vi "doma.vi"() -> ()   [LabVIEW 2017]
uses:
  <vilib>/userdefined/High Color/IMAQdx.ctl
  <vilib>/myRIO/Instrument Drivers/Onboard IO/DIO/typedefs/DIO Reference.ctl
  <vilib>/myRIO/Common/Instrument Driver Framework/Utilities/typedefs/myRIO Generic Hardware Reference.ctl
  <vilib>/myRIO/Common/Instrument Driver Framework/Utilities/typedefs/Hardware Version Enum.ctl
  <vilib>/myRIO/Common/Instrument Driver Framework/Utilities/typedefs/myRIO v1.0 Reference.ctl
  <vilib>/myRIO/Common/Instrument Driver Framework/Utilities/typedefs/Generic FPGA Reference.ctl
  <vilib>/myRIO/Common/Instrument Driver Framework/myRIO v1.0/DIO/typedefs/DIO Channels List.ctl
  <vilib>/myRIO/Common/Instrument Driver Framework/myRIO v1.0/DIO/typedefs/DIO Channels Enum.ctl
  <vilib>/userdefined/High Color/nirio_resource_hc.ctl
  <vilib>/myRIO/Common/Instrument Driver Framework/Utilities/vis/Is FPGA Ref Available.vi
  <vilib>/myRIO/Common/Instrument Driver Framework/myRIO v1.0/DIO/vis/myRIO v1.1 Open DIO.vi
  <vilib>/myRIO/Instrument Drivers/Onboard IO/DIO/vis/Write.vi
  <vilib>/myRIO/Common/Instrument Driver Framework/Utilities/vis/Validate Channels.vi
  <vilib>/myRIO/Common/Instrument Driver Framework/myRIO v1.0/DIO/vis/myRIO v1.0 Reserve DIO.vi
  <vilib>/myRIO/Common/Instrument Driver Framework/myRIO v1.0/Resource Manager/vis/myRIO v1.0 Reserve Channel List.vi
  <vilib>/myRIO/Common/Instrument Driver Framework/myRIO v1.0/DIO/vis/myRIO v1.0 Build MUX Configuration DIO.vi
  <vilib>/myRIO/Common/Instrument Driver Framework/myRIO v1.0/Resource Manager/vis/myRIO v1.0 Reserve Channel.vi
  <vilib>/myRIO/Common/Instrument Driver Framework/myRIO v1.0/Resource Manager/vis/myRIO v1.0 Unreserve Channel.vi
  <vilib>/myRIO/Common/Instrument Driver Framework/myRIO v1.0/Resource Manager/vis/myRIO v1.0 Create Configuration List.vi
  <vilib>/myRIO/Common/Instrument Driver Framework/myRIO v1.0/Resource Manager/vis/myRIO v1.0 Build Mutex Name.vi
  addres.vi
  <vilib>/Utility/VariantDataType/GetNumericInfo.vi
  <vilib>/Utility/error.llb/Error Cluster From Error Code.vi
  <vilib>/myRIO/Common/Instrument Driver Framework/myRIO v1.0/myRIO v1.1 Open.vi
  <vilib>/myRIO/Common/Instrument Driver Framework/Utilities/vis/IO Manager.vi
  <vilib>/myRIO/Common/Instrument Driver Framework/Utilities/vis/Configuration Manager.vi
  <vilib>/myRIO/Common/Instrument Driver Framework/myRIO v1.0/Resource Manager/vis/myRIO v1.0 Configure IO.vi
  <vilib>/myRIO/Common/Instrument Driver Framework/myRIO v1.0/myRIO v1.0 Close.vi
  <vilib>/myRIO/Common/Instrument Driver Framework/myRIO v1.0/DIO/vis/myRIO v1.0 Write DIO.vi
  <vilib>/myRIO/Express VI/Onboard Devices/LED/LED Express VI.xnode
  <vilib>/myRIO/Instrument Drivers/Onboard IO/DIO/vis/myRIO DIO Open.xnode
  <vilib>/vision/driver/NI_Vision_Acquisition_Software.lvlib
  <vilib>/myRIO/Instrument Drivers/Onboard IO/DIO/DIO.lvlib
panel:
  out "number":string
  out "color":string
  out "error out":errorcluster
  in  "error in":errorcluster
  out "Image":T1(plugin-control)
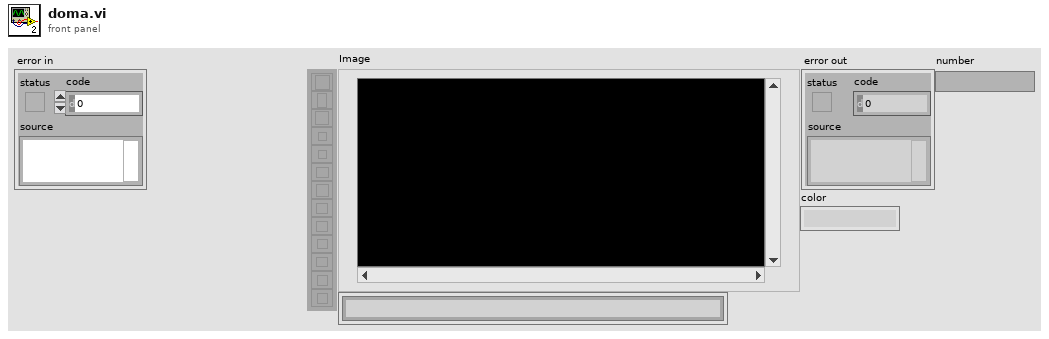
[diagram p1: front panel]
types:
  T1 = typedef "IMAQ Image.ctl" = refnum<image>
  T2 = typedef "IMAQdx.ctl" = refnum<k21>
  T3 = typedef "DIO.lvlib/DIO Reference.ctl" = cluster{"myRIO Reference":T4, "DIO Channels List":T8}
  T4 = typedef "myRIO Generic Hardware Reference.ctl" = cluster{"myRIO Model":T5, "myRIO Hardware Reference":T6}
  T5 = typedef "Hardware Version Enum.ctl" = enum16{"Unknown", "myRIO-1900", "myRIO-1950", "roboRIO", "NI ELVIS RIO CM"}
  T6 = typedef "myRIO v1.0 Reference.ctl" = cluster{"Generic FPGA Reference":T7, "Allow multiple opens":bool}
  T7 = typedef "Generic FPGA Reference.ctl" = refnum<k20>
  T8 = typedef "DIO Channels List.ctl" = T9[]
  T9 = typedef "DIO Channels Enum.ctl" = enum16{"Not Connected", "C/DIO0", "C/DIO1", "C/DIO2", "C/DIO3", "C/DIO4", "C/DIO5", "C/DIO6", "C/DIO7", "A/DIO0", "A/DIO1", "A/DIO2", "A/DIO3", "A/DIO4", "A/DIO5", "A/DIO6", "A/DIO7", "A/DIO8", "A/DIO9", "A/DIO10", "A/DIO11", "A/DIO12", "A/DIO13", "A/DIO14", "A/DIO15", "B/DIO0", "B/DIO1", "B/DIO2", "B/DIO3", "B/DIO4", "B/DIO5", "B/DIO6", "B/DIO7", "B/DIO8", "B/DIO9", "B/DIO10", "B/DIO11", "B/DIO12", "B/DIO13", "B/DIO14", "B/DIO15", "LED0", "LED1", "LED2", "LED3", "Button0", "DIO/DIO0", "DIO/DIO1", "DIO/DIO2", "DIO/DIO3", "DIO/DIO4", "DIO/DIO5", "DIO/DIO6", "DIO/DIO7", "DIO/DIO8", "DIO/DIO9", "SPI/CS0", "SPI/CS1", "SPI/CS2", "SPI/CS3", "LED RADIO (Green)", "LED RADIO (Red)", "LED COMM (Green)", "LED COMM (Red)", "LED MODE (Green)", "LED MODE (Red)"}
  T10 = typedef "nirio_resource_hc.ctl" = tag
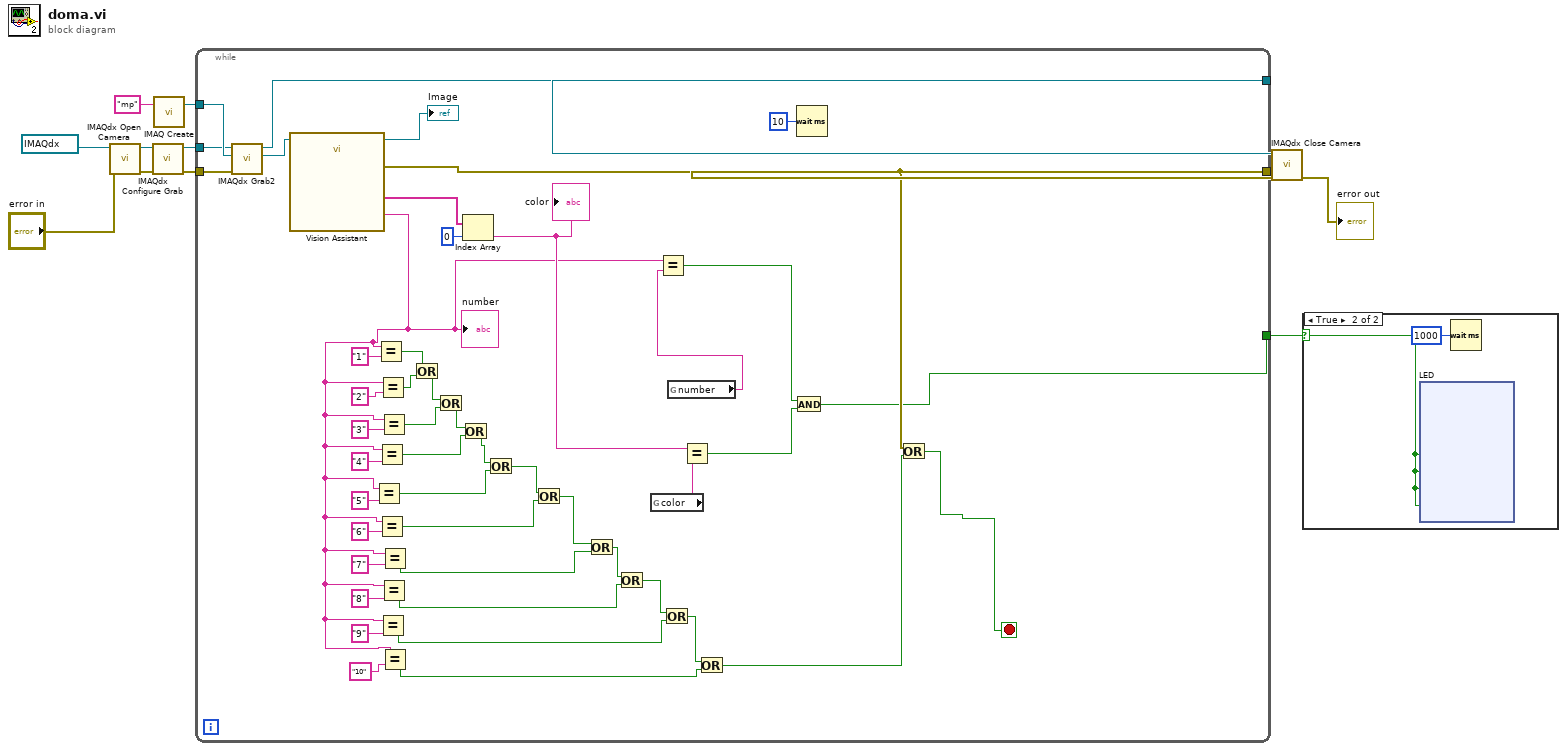
[diagram p0: block diagram]
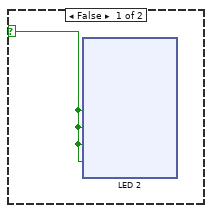
[diagram p2: hidden frame]
diagram:
  n1 = call <vilib>:"IMAQdx Open Camera.vi"("error in"="error in", "Session In"=T2 "cam0") -> ("error out"=w6:errorcluster, "Session Out"=w9:T2)  [unwired: 8 in]
  n2 = call <vilib>:"IMAQdx Configure Grab.vi"("error in"=w6, "Session In"=w9) -> ("error out"=w7:errorcluster, "Session Out"=w10:T2)  [unwired: 8 in]
  n3 = call "IMAQ Create"("Image Name"="mp") -> ("New Image"=w8:T1)  [unwired: 4 in, 1 out]
  n4 = while {
    tunnel: w7 -> [w59]
    tunnel: w8 -> [w58]
    tunnel: w10 -> [w57]
    tunnel: [w56] -> w11
    tunnel: [w45] -> w12
    tunnel: [w13] -> w1
    stop <- w15 stop-if-true
    n5 = call <vilib>:"IMAQdx Grab2.vi"("error in"=w59, "Image In"=w58, "Session In"=w57) -> ("Image Out"=w54:T1, "Session Out"=w56:T2)  [unwired: 5 in, 2 out]
    n6 = call "Vision Assistant"("Image In"=w54) -> ("Image Out"=→"Image":T1, "Classes (Color Classification 1)"=w52:string[], "String (OCR/OCV 1)"=w16:string, "error out"=w45:errorcluster)  [unwired: 23 in]
    "number" <- w16
    n7 = Equal?(x=w16, y="5") -> (x = y?=w34:bool)
    n8 = Equal?(x=w16, y="1") -> (x = y?=w27:bool)
    n9 = Equal?(x=w16, y="4") -> (x = y?=w32:bool)
    n10 = Equal?(x=w16, y="6") -> (x = y?=w36:bool)
    n11 = Equal?(x=w16, y="2") -> (x = y?=w28:bool)
    n12 = Equal?(x=w16, y="9") -> (x = y?=w42:bool)
    n13 = Equal?(x=w16, y="3") -> (x = y?=w30:bool)
    n14 = Equal?(x=w16, y="8") -> (x = y?=w39:bool)
    n15 = Equal?(x=w16, y="7") -> (x = y?=w38:bool)
    n16 = Equal?(x=w16, y="10") -> (x = y?=w44:bool)
    n17 = Or(x=w27, y=w28) -> (x .or. y?=w29:bool)
    n18 = Or(x=w29, y=w30) -> (x .or. y?=w31:bool)
    n19 = Or(x=w31, y=w32) -> (x .or. y?=w33:bool)
    n20 = Index Array(array=w52, index=0) -> (element=w48:string)
    "color" <- w48
    n21 = Or(x=w33, y=w34) -> (x .or. y?=w35:bool)
    n22 = Or(x=w35, y=w36) -> (x .or. y?=w37:bool)
    n23 = Or(x=w37, y=w38) -> (x .or. y?=w40:bool)
    n24 = Or(x=w40, y=w39) -> (x .or. y?=w41:bool)
    n25 = global read "addres.vi" "color"() -> (w49:string)
    n26 = Or(x=w41, y=w42) -> (x .or. y?=w43:bool)
    n27 = global read "addres.vi" "number"() -> (w50:string)
    n28 = Equal?(x=w16, y=w50) -> (x = y?=w46:bool)
    n29 = Equal?(x=w48, y=w49) -> (x = y?=w47:bool)
    n30 = Or(x=w43, y=w44) -> (x .or. y?=w14:bool)
    n31 = And(x=w46, y=w47) -> (x .and. y?=w13:bool)
    n32 = Wait (ms)(milliseconds to wait=u32 10) -> ()  [unwired: 1 out]
    n33 = Or(x=w45, y=w14) -> (x .or. y?=w15:bool)
  }
  n34 = call <vilib>:"IMAQdx Close Camera.vi"("error in"=w12, "Session In"=w11) -> ("error out"=→"error out":errorcluster)  [unwired: 9 in]
  n35 = case shown="True" w1 {
    selector: w1 -> [w60 w99]
    frame False {
      n36 = xnode "LED 2"("LED0"=w60, "LED1"=w60, "LED2"=w60, "LED3"=w60) -> ()  [unwired: 1 in, 1 out]
    }
    frame True {
      n37 = xnode "LED"("LED0"=w99, "LED1"=w99, "LED2"=w99, "LED3"=w99) -> ()  [unwired: 1 in, 1 out]
      n38 = Wait (ms)(milliseconds to wait=u32 1000) -> ()  [unwired: 1 out]
    }
  }
